vi "rcm_gain_adjust.vi"(7 "Reset":bool, 9 "Goal tip pos":sgl[](array[numeric]), 10 "Goal pose (handle basis) in":T12, 11 "Parameters":T1={"Stimulus"={"Type"=enum."Off", "Phase"=0.0, "Amplitude"=[], "Injection point"=enum."Total pose", "Closed loop"=FALSE, "Offset"=[], "Tip -> world"=FALSE, "Frequency"=0.0, "Length"=0.0}, "Goal Filter A"={"Speedup max"=0.0, "Speedup thresh"=0.0, "Speedup nonlin"=0.0, "Filters"=[]}, "Mode controls"={"Hold"=FALSE, "Cancellation"=FALSE, "Goal filter"=FALSE, "Trigger"=FALSE}, "Manipulator type"=enum."Current piezo", "Manipulator calibration"={"Tool offsets"=[[0.0, 0.0, 36200.0]], "Handle light calibration"=[], "Base pivots"=[], "Output pivots"=[], "Length center"=0.0, "Workspace height"=[], "Workspace diameter"=[0.0, 0.0, 36200.0], "Stack travel"=400.0, "Saturation pos"=375.0, "Inverse filters"=[], "Strut length"=0.0}, "Network"={"Remote Host"="", "Send Status"=FALSE, "Send Port"=0, "Recv Commands"=FALSE, "Recv Port"=0}, "Goal Filter B"={"Speedup max"=0.0, "Speedup thresh"=0.0, "Speedup nonlin"=0.0, "Filters"=[]}, "Cancellation"={"KP"={"XY"=0.0, "Rxy"=0.0, "Z"=0.0, "Rz"=0.0}, "KI"=0.0, "KD"={"XY"=0.0, "Rxy"=0.0, "Z"=0.0, "Rz"=0.0}, "Max vel"=20.0, "Max acc"=0.001, "Int error limit"=3.0, "RCM gain"=0.0, "Bypass"=FALSE, "Degraded gain"=0.0}, "Transition time"=0.0, "Estimation"={"Link"={"Measure noise"=[], "Process noise"=[], "Alt process noise"=[], "Alt turnoff cycles"=20, "Innovation limit"=[], "Residue threshold"=0.0, "Enable"=FALSE}, "Handle"={"Measure noise"=[], "Process noise"=[], "State limits"=[], "Innovation limit"=[], "Prediction Lookahead"=0.0, "Enable"=FALSE}}} {"Transition time" format="%_3f"; "Cancellation"."Degraded gain" min=0 max=1 step=0.1 format="%#_3p"; "Cancellation"."RCM gain" min=0 max=1 step=0.1 format="%#_3p"; "Cancellation"."KD"."Rz" min=-1 max=1 step=0.01 format="%#_3p"; "Cancellation"."KD"."Rxy" min=-1 max=1 step=0.01 format="%#_3p"; "Cancellation"."KD"."Z" min=-1 max=1 step=0.01 format="%#_3p"; "Cancellation"."KD"."XY" min=-1 max=1 step=0.01 format="%#_3p"; "Cancellation"."KI" min=0 max=1 step=0.01 format="%#_3p"; "Cancellation"."KP"."Rz" min=-1 max=1 step=0.01 format="%#_3p"; "Cancellation"."KP"."Rxy" min=-1 max=1 step=0.01 format="%#_3p"; "Cancellation"."KP"."Z" min=-1 max=1 step=0.01 format="%#_3p"; "Cancellation"."KP"."XY" min=-1 max=1 step=0.01 format="%#_3p"; "Cancellation"."Max acc" format="%#_3p"; "Goal Filter B"."Filters"."V limit range" format="%_3p"; "Goal Filter B"."Filters"."V limit" format="%_3p"; "Goal Filter B"."Filters"."Upper Q" format="%_3f"; "Goal Filter B"."Filters"."Upper Fc" format="%_3p"; "Goal Filter B"."Filters"."Lower Q" format="%_3f"; "Goal Filter B"."Filters"."Scale factor" format="%_3f"; "Goal Filter B"."Filters"."Lower Fc" format="%_3p"; "Goal Filter B"."Speedup nonlin" format="%_3p"; "Goal Filter B"."Speedup thresh" format="%_3p"; "Goal Filter B"."Speedup max" format="%_3p"; "Manipulator calibration"."Strut length" format="%#_4p"; "Manipulator calibration"."Saturation pos" format="%#.1f"; "Manipulator calibration"."Stack travel" format="%#.1f"; "Manipulator calibration"."Length center" format="%#_4p"; "Manipulator calibration"."Output pivots" format="%#_6f"; "Manipulator calibration"."Base pivots" format="%#_6f"; "Manipulator calibration"."Handle light calibration" format="%#.1f"; "Goal Filter A"."Filters"."V limit range" format="%_3p"; "Goal Filter A"."Filters"."V limit" format="%_3p"; "Goal Filter A"."Filters"."Upper Q" format="%_3f"; "Goal Filter A"."Filters"."Upper Fc" format="%_3p"; "Goal Filter A"."Filters"."Lower Q" format="%_3f"; "Goal Filter A"."Filters"."Scale factor" format="%_3f"; "Goal Filter A"."Filters"."Lower Fc" format="%_3p"; "Goal Filter A"."Speedup nonlin" format="%_3p"; "Goal Filter A"."Speedup thresh" format="%_3p"; "Goal Filter A"."Speedup max" format="%_3p"; "Stimulus"."Length" min=0.0 max=100.0 step=100.0 format="%#_4p"; "Stimulus"."Frequency" min=0.0 step=100.0 format="%#_4g"; "Stimulus"."Offset" format="%#_3p"; "Stimulus"."Amplitude" format="%#_3p"; "Stimulus"."Phase" min=-180.0 max=360.0 step=100.0 format="%#.2f"}) -> (3 "Goal pose (handle basis) out":T12)   [LabVIEW 2014]
uses:
  <vilib>/Analysis/Matrix/Datatypes/RealMatrix.ctl
  testing/Micron params.ctl
  testing/stimulus.ctl
  testing/injection_point.ctl
  goal_loop_parms.ctl
  testing/mode_conrols.ctl
  testing/manipulator_cal.ctl
  asap/labview/testing/probe_calibration.ctl
  host/network_params.ctl
  cancellation/sq_control_params.ctl
  cancellation/decoupled_gain.ctl
  cancellation/estimation_controls.ctl
  <vilib>/Analysis/baseanly.llb/A x Vector.vi
  <vilib>/Analysis/Matrix/Numeric/Conversions/Array To Matrix - RA2.vi
  <vilib>/Analysis/Matrix/Numeric/Multiply/Multiply - RM,R.vi
  <vilib>/Analysis/Matrix/Numeric/Multiply/Multiply - R,RM.vi
  <vilib>/Analysis/Matrix/Numeric/Add/Add - RM,RM.vi
  <vilib>/Analysis/NI_AALBase.lvlib
  <vilib>/Analysis/Matrix/NI_Matrix.lvlib
panel:
  in  "Q":dbl=0.7
  in  "Fc":dbl=70.0
  # "Parameters for lowpass filter on the RCM gain path."
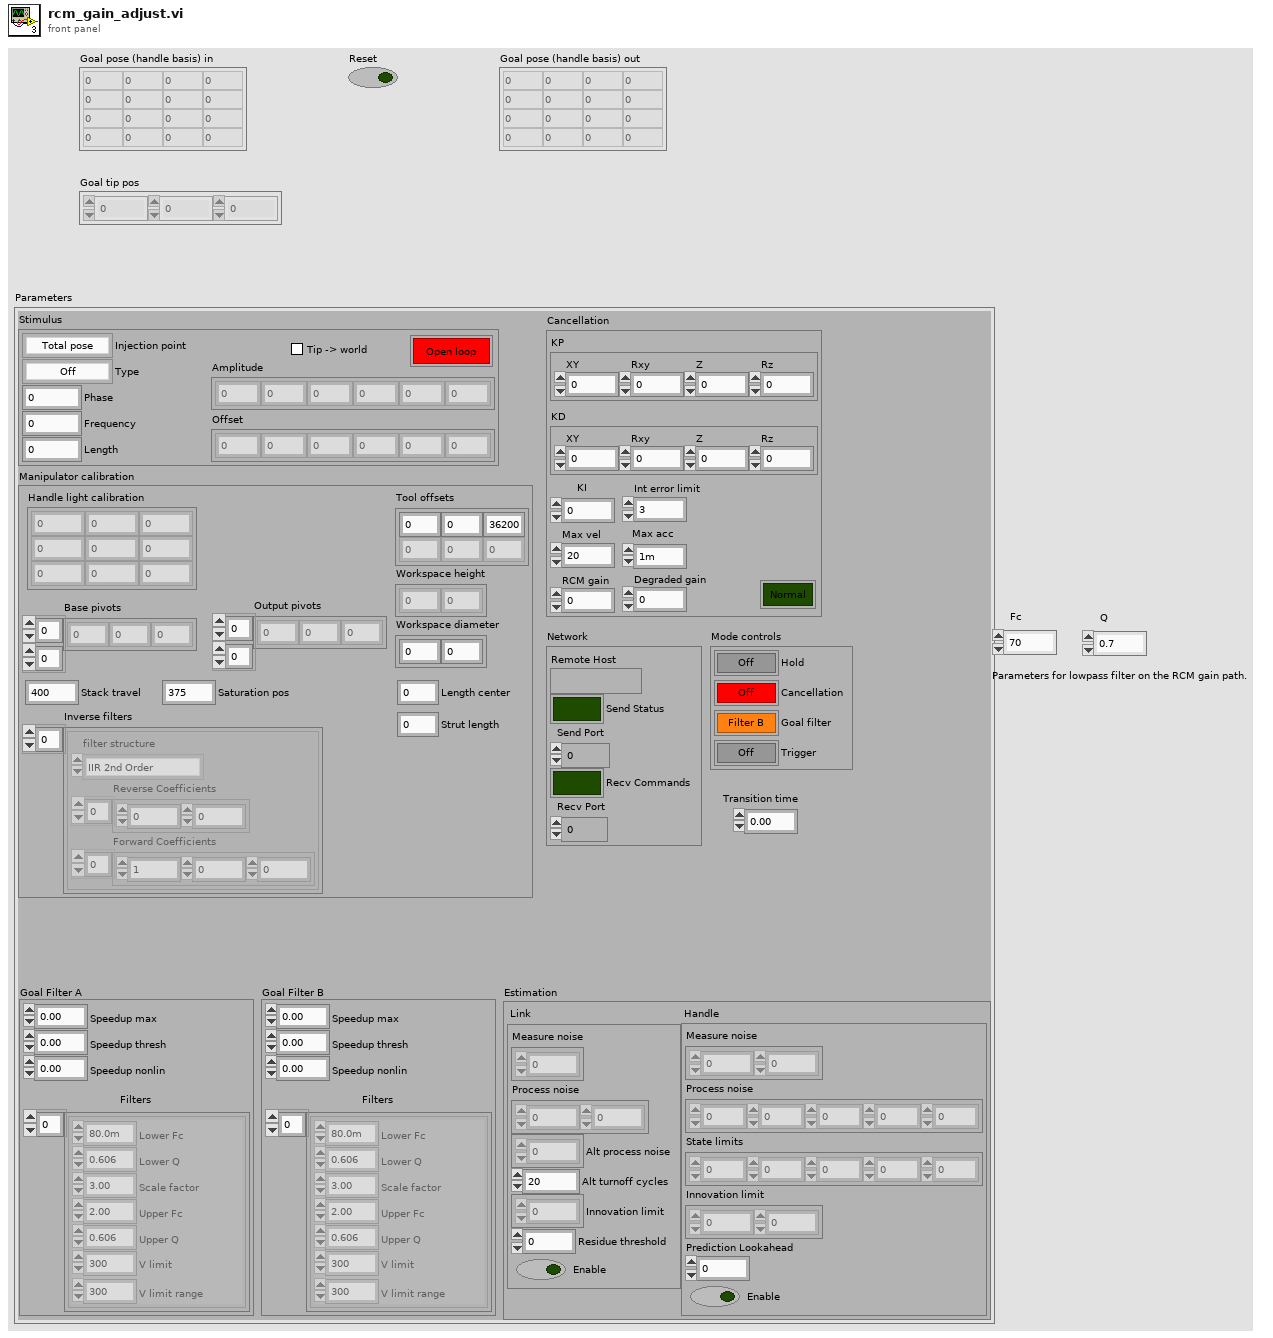
[diagram p1: front panel]
types:
  T1 = typedef "Micron params.ctl" = cluster{"Stimulus":T2, "Goal Filter A":T4, "Mode controls":T5, "Manipulator type":enum16{"Current piezo", "Voltage piezo"}, "Manipulator calibration":T6, "Network":T8, "Goal Filter B":T4, "Cancellation":T9, "Transition time":sgl, "Estimation":T11}
  T2 = typedef "stimulus.ctl" = cluster{"Type":enum16{"Off", "Step", "Sine", "Triangle", "Arbitrary"}, "Phase":dbl, "Amplitude":sgl[], "Injection point":T3, "Closed loop":bool, "Offset":sgl[], "Tip -> world":bool, "Frequency":dbl, "Length":dbl}
  T3 = typedef "injection_point.ctl" = enum16{"Total pose", "V limiter", "Goal ", "Link position", "KF link position", "Inverse kin", "Link goal", "Link error", "Controller", "Output", "Drive", "Light"}
  T4 = typedef "goal_loop_parms.ctl" = cluster{"Speedup max":sgl, "Speedup thresh":sgl, "Speedup nonlin":sgl, "Filters":cluster{"Lower Fc":sgl, "Lower Q":sgl, "Scale factor":sgl, "Upper Fc":sgl, "Upper Q":sgl, "V limit":sgl, "V limit range":sgl}[]}
  T5 = typedef "mode_conrols.ctl" = cluster{"Hold":bool, "Cancellation":bool, "Goal filter":bool, "Trigger":bool}
  T6 = typedef "manipulator_cal.ctl" = cluster{"Tool offsets":sgl[][], "Handle light calibration":T7, "Base pivots":sgl[][], "Output pivots":sgl[][], "Length center":sgl, "Workspace height":sgl[], "Workspace diameter":sgl[], "Stack travel":sgl, "Saturation pos":sgl, "Inverse filters":cluster{"filter structure":enum32{"IIR 2nd Order", "IIR 4th Order"}, "Reverse Coefficients":dbl[], "Forward Coefficients":dbl[]}[], "Strut length":sgl}
  T7 = typedef "probe_calibration.ctl" = sgl[][]
  T8 = typedef "network_params.ctl" = cluster{"Remote Host":string, "Send Status":bool, "Send Port":u16, "Recv Commands":bool, "Recv Port":u16}
  T9 = typedef "sq_control_params.ctl" = cluster{"KP":T10, "KI":sgl, "KD":T10, "Max vel":sgl, "Max acc":sgl, "Int error limit":sgl, "RCM gain":sgl, "Bypass":bool, "Degraded gain":sgl}
  T10 = typedef "decoupled_gain.ctl" = cluster{"XY":sgl, "Rxy":sgl, "Z":sgl, "Rz":sgl}
  T11 = typedef "estimation_controls.ctl" = cluster{"Link":cluster{"Measure noise":dbl[], "Process noise":dbl[], "Alt process noise":dbl[], "Alt turnoff cycles":i32, "Innovation limit":dbl[], "Residue threshold":dbl, "Enable":bool}, "Handle":cluster{"Measure noise":dbl[], "Process noise":dbl[], "State limits":dbl[], "Innovation limit":dbl[], "Prediction Lookahead":sgl, "Enable":bool}}
  T12 = typedef "NI_Matrix.lvlib/RealMatrix.ctl" = dbl[][]
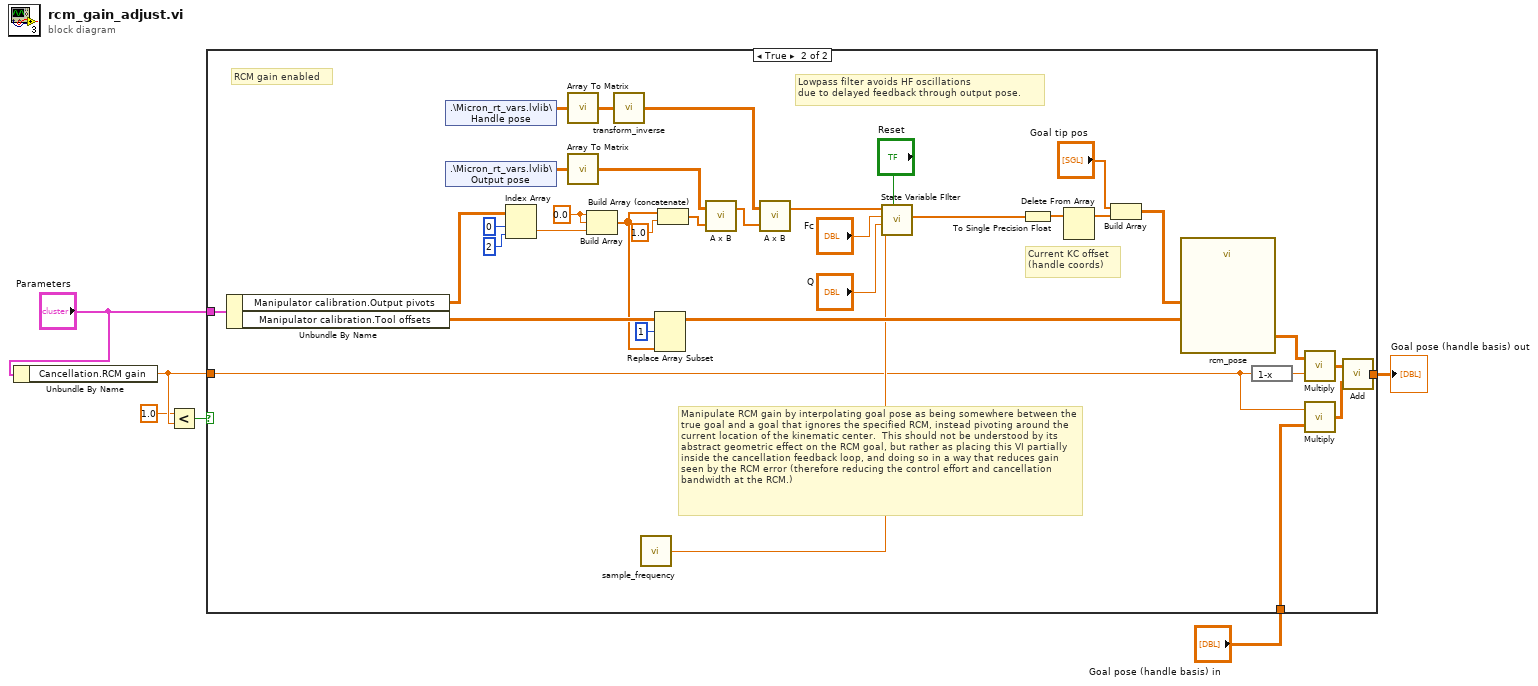
[diagram p0: block diagram]
diagram:
  n1 = Unbundle By Name("Parameters") -> ("Cancellation.RCM gain"=w3:sgl)
  n2 = Less?(x=sgl 1.0, y=w3) -> (x < y?=w1:bool)
  n3 = case shown="True" w1 {
    tunnel: "Goal pose (handle basis) in" -> [w7 w18]
    tunnel: [w7 w16] -> w5
    tunnel: "Parameters" -> [_ w9]
    tunnel: w3 -> [_ w8]
    frame False {
      # "Gain of 1 means off."
    }
    frame True {
      w42 = sgl 0.0 ("Numeric")
      # "RCM gain enabled"
      # "Lowpass filter avoids HF oscillations\ndue to delayed feedback through output pose."
      # "Current KC offset\n(handle coords)"
      # "Manipulate RCM gain by interpolating goal pose as being somewhere between the true goal and a goal that ignores the specified RCM, instead pivoting around the current location of the kinematic center.  This should not be understood by its abstract geometric effect on the RCM goal, but rather as placing this VI partially inside the cancellation feedback loop, and doing so in a way that reduces gain seen by the RCM error (therefore reducing the control effort and cancellation bandwidth at the RCM.)"
      n4 = Unbundle By Name(w9) -> ("Manipulator calibration.Output pivots"=w22:sgl[][], "Manipulator calibration.Tool offsets"=w41:sgl[][])
      n5 = shared-variable ".\\Micron_rt_vars.lvlib\\Handle pose"() -> (w24:sgl[][])  [unwired: 2 out]
      n6 = shared-variable ".\\Micron_rt_vars.lvlib\\Output pose"() -> (w28:sgl[][])  [unwired: 2 out]
      n7 = Index Array(array=w22, index (row)=0 ("disabled index (row)"), index (col)=2 ("disabled index (col)")) -> (element=w37:sgl)
      n8 = call-poly <vilib>:"Array To Matrix.vi"("Real 2D Array"=w24) -> ("Real Matrix"=w25:T12)
      n9 = call-poly <vilib>:"Array To Matrix.vi"("Real 2D Array"=w28) -> ("Real Matrix"=w30:T12)
      n10 = Build Array(w42, w42, w37) -> (w26:sgl[])
      n11 = call "transform_inverse.vi"("Transform"=w25) -> ("Inverse transform"=w23:T12)
      n12 = call "sample_frequency.vi"() -> ("Sample frequency"=w12:dbl)
      n13 = Replace Array Subset(array=w41, new element=w26, index (row)=1) -> (w36:sgl[][])  [unwired: 1 in]
      n14 = Build Array (concatenate)(w26, sgl 1.0) -> (w31:sgl[])
      n15 = call-poly <vilib>:"A x B.vi"("Vector"=w31, "A"=w30) -> ("A x Vector"=w27:dbl[])  [unwired: 1 out]
      n16 = call-poly <vilib>:"A x B.vi"("Vector"=w27, "A"=w23) -> ("A x Vector"=w15:dbl[])  [unwired: 1 out]
      n17 = call "State Variable FIlter.vi"("initialize"="Reset", "Fs"=w12, "Q"="Q", "Fc"="Fc", "x"=w15) -> ("Lowpass"=w10:dbl[])  [unwired: 4 in, 2 out]
      n18 = To Single Precision Float(number=w10) -> (single precision float=w29:sgl[])
      n19 = Delete From Array(array=w29) -> (array with subset deleted=w20:sgl[])  [unwired: 2 in, 1 out]
      n20 = Build Array("Goal tip pos", w20) -> (w19:sgl[][])
      n21 = call "rcm_pose.vi"("Goal positions"=w19, "Nominal positions"=w36) -> ("Goal pose (handle basis)"=w17:T12)  [unwired: 9 in]
      n22 = expression code="1-x"(w8) -> (w33:sgl)
      n23 = call-poly <vilib>:"Multiply.vi"("Real Scalar c"=w33, "Real Matrix A"=w17) -> ("A * c"=w35:T12)
      n24 = call-poly <vilib>:"Multiply.vi"("Real Matrix A"=w18, "Real Scalar c"=w8) -> ("c * A"=w34:T12)
      n25 = call-poly <vilib>:"Add.vi"("Real Matrix B"=w34, "Real Matrix A"=w35) -> ("A + B"=w16:T12)
    }
  }
  "Goal pose (handle basis) out" <- w5
